vi "Data Entry.vi"(8 "error in (no error)":errorcluster, 10 "Data":T1 {"offset" format="%.3g"}, 11 "Byte Stream File in":refnum<file>) -> (0 "error out":errorcluster, 3 "Byte Stream File out":refnum<file>)   [LabVIEW 2018, in "Logging.lvlib"]
uses:
  Logging.lvlib
  Controls/Acquired Data.ctl
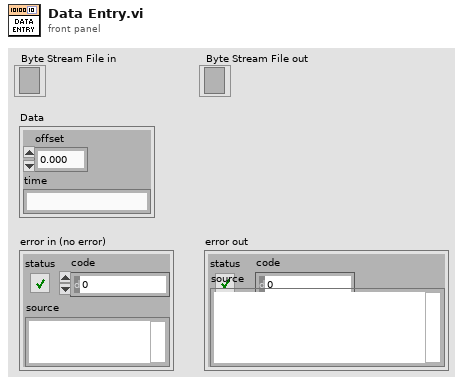
[diagram p1: front panel]
types:
  T1 = typedef "Acquired Data.ctl" = cluster{"offset":dbl, "time":string}
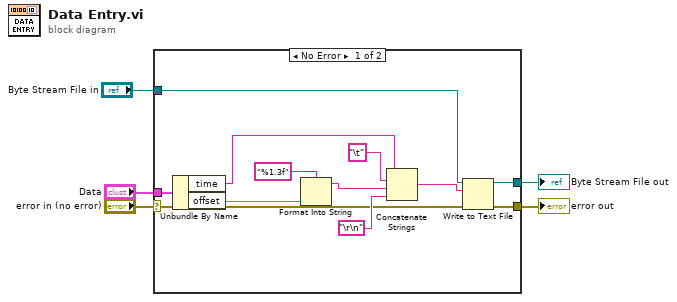
[diagram p0: block diagram]
diagram:
  n1 = case shown="No Error" "error in (no error)" {
    selector: "error in (no error)" -> [w6 w18]
    tunnel: "Data" -> [w17 _]
    tunnel: [w16 w18] -> w4
    tunnel: [w15 w19] -> w3
    tunnel: "Byte Stream File in" -> [w14 w19]
    frame No Error {
      n2 = Unbundle By Name(w17) -> ("time"=w13:string, "offset"=w7:dbl)
      n3 = Format Into String(format string="%1.3f", w7) -> (resulting string=w10:string)  [unwired: 2 in, 1 out]
      n4 = Concatenate Strings(w13, "\t" ("format string"), w10, "\r\n") -> (w12:string)
      n5 = Write to Text File(file (use dialog)=w14, text=w12, error in=w6) -> (refnum out=w15:refnum<file>, error out=w16:errorcluster)  [unwired: 1 in, 1 out]
    }
    frame Error {
    }
  }
  "error out" <- w4
  "Byte Stream File out" <- w3
